vi "TemperatureWarning(SubVI).vi"(8 "error in (no error)":errorcluster, 11 "Weather In":T1={"Current Temperature"=0.0, "Max Temperature"=0.0, "Min Temperature"=0.0, "Warning?"=FALSE, "Warning Text"="No Warning"}) -> (0 "error out":errorcluster, 3 "Weather Out":T1={"Current Temperature"=0.0, "Max Temperature"=0.0, "Min Temperature"=0.0, "Warning?"=FALSE, "Warning Text"="No Warning"})   [LabVIEW 2021]
doc: "Temperature Warining When Too Hot or Cold"
uses:
  WeatherData.ctl
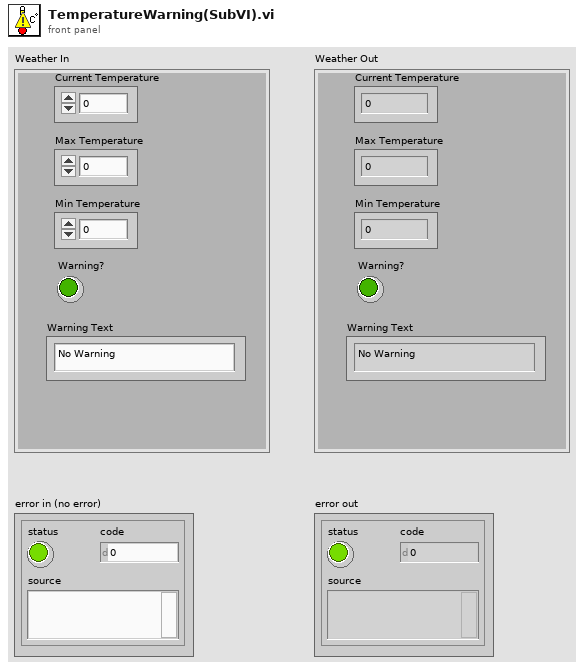
[diagram p1: front panel]
types:
  T1 = typedef "WeatherData.ctl" = cluster{"Current Temperature":dbl, "Max Temperature":dbl, "Min Temperature":dbl, "Warning?":bool, "Warning Text":string}
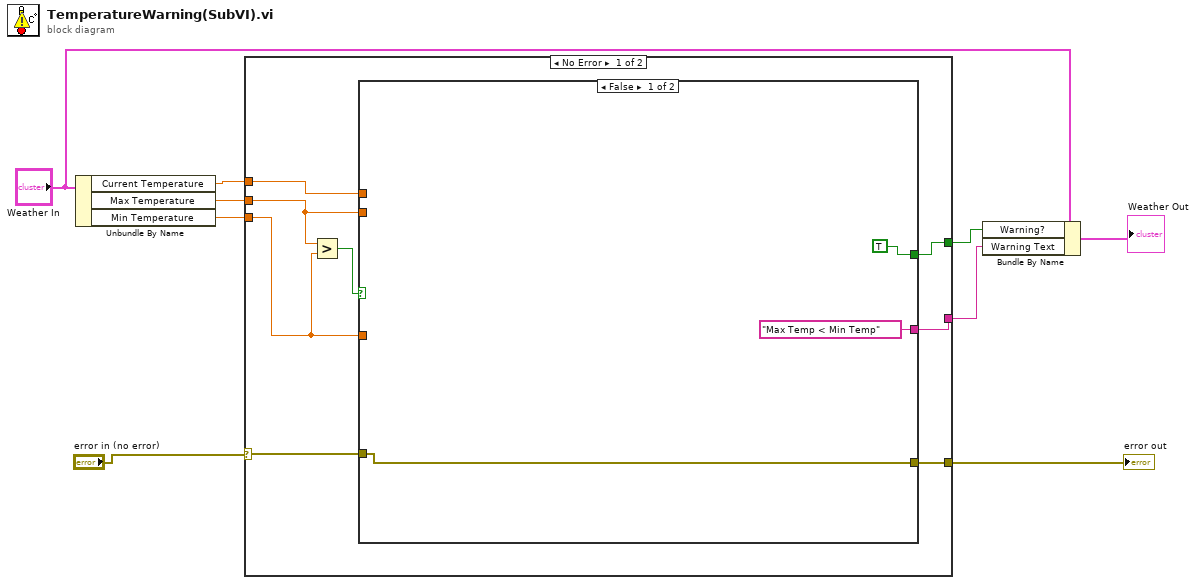
[diagram p0: block diagram]
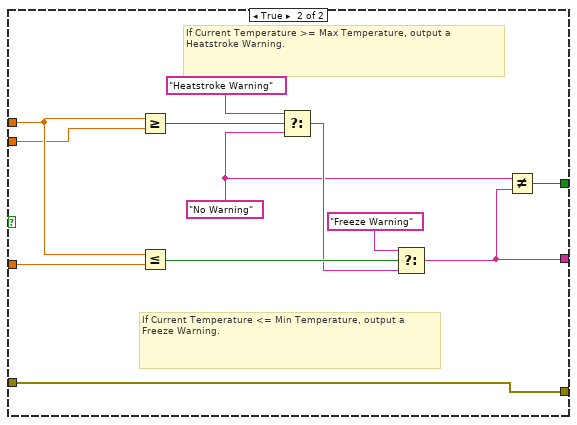
[diagram p2: hidden frame]
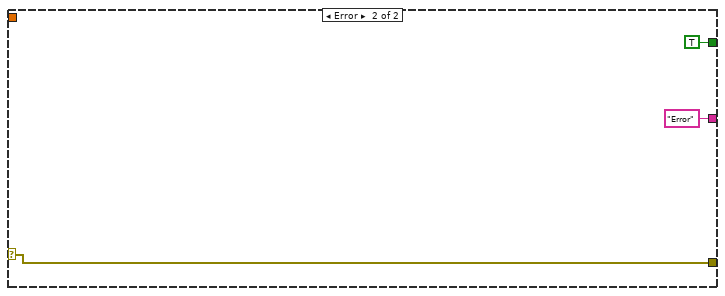
[diagram p3: hidden frame]
diagram:
  n1 = Unbundle By Name("Weather In") -> ("Current Temperature"=w1:dbl, "Max Temperature"=w2:dbl, "Min Temperature"=w3:dbl)
  n2 = case shown="No Error" "error in (no error)" {
    selector: "error in (no error)" -> [w10 w33]
    tunnel: w1 -> [w17 _]
    tunnel: w2 -> [w14 _]
    tunnel: w3 -> [w13 _]
    tunnel: [w16 TRUE] -> w5
    tunnel: [w15 "Error" ("f")] -> w6
    tunnel: [w11 w33] -> w9
    frame No Error {
      n3 = Greater?(x=w14, y=w13) -> (0:w12:bool)
      n4 = case shown="False" w12 {
        tunnel: w17 -> [_ w26]
        tunnel: w14 -> [_ w25]
        tunnel: w13 -> [_ w24]
        tunnel: [TRUE w23] -> w16
        tunnel: ["Max Temp < Min Temp" ("f") w22] -> w15
        tunnel: [w18 w21] -> w11
        tunnel: w10 -> [w18 w21]
        frame False {
        }
        frame True {
          w27 = "No Warning" ("f")
          # "If Current Temperature >= Max Temperature, output a Heatstroke Warning."
          # "If Current Temperature <= Min Temperature, output a Freeze Warning."
          n5 = Greater Or Equal?(x=w26, y=w25) -> (x >= y?=w32:bool)
          n6 = Less Or Equal?(x=w26, y=w24) -> (x <= y?=w29:bool)
          n7 = Select(t="Heatstroke Warning", s=w32, f=w27) -> (s? t:f=w28:string)
          n8 = Select(t="Freeze Warning", s=w29, f=w28) -> (s? t:f=w22:string)
          n9 = Not Equal?(x=w27, y=w22) -> (x != y?=w23:bool)
        }
      }
    }
    frame Error {
    }
  }
  "error out" <- w9
  n10 = Bundle By Name(cluster="Weather In", "Warning?"=w5, "Warning Text"=w6) -> (→"Weather Out":T1)
